vi "sub_init-floodf-ill.vi"() -> (3 "occupancy_map":T1)   [LabVIEW 2019]
uses:
  <vilib>/Analysis/Matrix/Datatypes/RealMatrix.ctl
  Ctrl/cmd_common.ctl
  <vilib>/Analysis/Matrix/Numeric/Conversions/Array To Matrix - RA2.vi
  <vilib>/Analysis/Matrix/NI_Matrix.lvlib
panel:
  out "prev ix/iv":cluster{"center x":i32, "center y":i32}
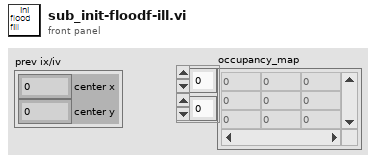
[diagram p1: front panel]
types:
  T1 = typedef "NI_Matrix.lvlib/RealMatrix.ctl" = dbl[][]
  T2 = typedef "cmd_common.ctl" = enum16{"read", "write"}
  T3 = cluster{"xy_resolution":dbl, "EXTEND_AREA":dbl, "MAX_RANGE":dbl, "NP":u32, "NTh":u32, "Q":T1, "R":T1, "Q_sim":T1, "R_sim":T1, "rf_id":cluster{"x":dbl, "y":dbl}[], "map x size":u32, "map y size":u32, "map x center":u32, "map y center":u32}
  T4 = cluster{"ox":dbl[], "oy":dbl[], "occupancy map":T1, "x_true":T1, "u":T1, "z":T1, "PEst":T1, "min x":dbl, "min y":dbl, "max x":dbl, "max y":dbl, "yw":i32, "xw":i32, "center x":i32, "center y":i32}
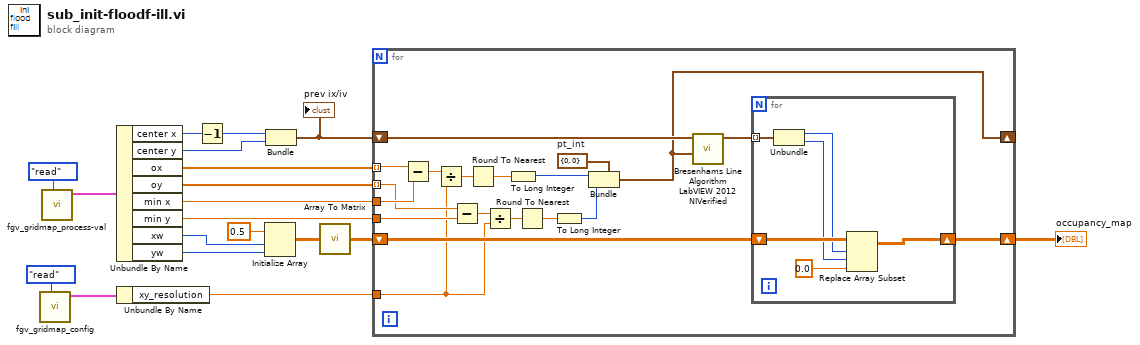
[diagram p0: block diagram]
diagram:
  n1 = call "fgv_gridmap_config.vi"("cmd"=cmd_common."read") -> ("pf-val out"=w16:T3)  [unwired: 10 in]
  n2 = call "fgv_gridmap_process-val.vi"("cmd"=cmd_common."read") -> ("p-val  2"=w18:T4)  [unwired: 10 in]
  n3 = Unbundle By Name(w18) -> ("center x"=w15:i32, "center y"=w8:i32, "ox"=w14:dbl[], "oy"=w13:dbl[], "min x"=w12:dbl, "min y"=w10:dbl, "xw"=w6:i32, "yw"=w5:i32)
  n4 = Unbundle By Name(w16) -> ("xy_resolution"=w11:dbl)
  n5 = Decrement(x=w15) -> (x-1=w9:i32)
  n6 = Initialize Array(0.5 ("element"), w6, w5) -> (w3:dbl[][])
  n7 = Bundle(w9, "center y"=w8) -> (w7:cluster{i32, "center y":i32})  [unwired: 1 in]
  "prev ix/iv" <- w7
  n8 = call-poly <vilib>:"Array To Matrix.vi"("Real 2D Array"=w3) -> ("Real Matrix"=w2:T1)
  n9 = for {
    tunnel: w14 -> [w38] mode=indexing
    tunnel: w13 -> [w32] mode=indexing
    tunnel: w12 -> [w37]
    tunnel: w11 -> [w22]
    tunnel: w10 -> [w31]
    shift-right: [w23] -> w1
    shift-left: w2 -> [w24]
    shift-right: [w20] -> _
    shift-left: w7 -> [w21]
    w26 = cluster{"x":i32, "y":i32} {"x"=0, "y"=0}  # pt_int
    n10 = Subtract(x=w38, y=w37) -> (x-y=w36:dbl)
    n11 = Divide(x=w36, y=w22) -> (x/y=w35:dbl)
    n12 = Subtract(x=w32, y=w31) -> (x-y=w33:dbl)
    n13 = Round To Nearest(number=w35) -> (nearest integer value=w30:dbl)
    n14 = Divide(x=w33, y=w22) -> (x/y=w34:dbl)
    n15 = To Long Integer(number=w30) -> (32bit integer=w27:i32)
    n16 = Round To Nearest(number=w34) -> (nearest integer value=w29:dbl)
    n17 = To Long Integer(number=w29) -> (32bit integer=w28:i32)
    n18 = Bundle(cluster=w26, "x"=w27, "y"=w28) -> (w20:cluster{"x":i32, "y":i32})
    n19 = call "Bresenhams Line Algorithm LabVIEW 2012 NIVerified.vi"("End"=w20, "Start"=w21) -> ("Line Points"=w25:cluster{"X":i32, "Y":i32}[])  [unwired: 8 in, 1 out]
    n20 = for {
      tunnel: w25 -> [w42] mode=indexing
      shift-right: [w43] -> w23
      shift-left: w24 -> [w44]
      n21 = Unbundle(w42) -> ("X"=w41:i32, "Y"=w40:i32)
      n22 = Replace Array Subset(array=w44, new element=0.0 ("new element/submatrix"), index (row)=w41, index (col)=w40) -> (w43:T1)
    }
  }
  "occupancy_map" <- w1
